vi "LvMPDC_SUB_SendCmdAndRecvReply_2.vi"(6 "timeout_ms":i32=3000, 8 "error in (no error)":errorcluster, 9 "ReadBytes":i32=10240, 10 "Command":string="ping", 11 "Connect ID":refnum<k5>) -> (0 "error out":errorcluster, 2 "Reply":string, 3 "Connect ID out":refnum<k5>)   [LabVIEW 2012]
panel:
  out "Recv String":string
  # "LvMPDC:: Send Command and ReceiveReply"
  # "Replyは、\n末尾の\"OK\\n\"を取り除いた文字列"
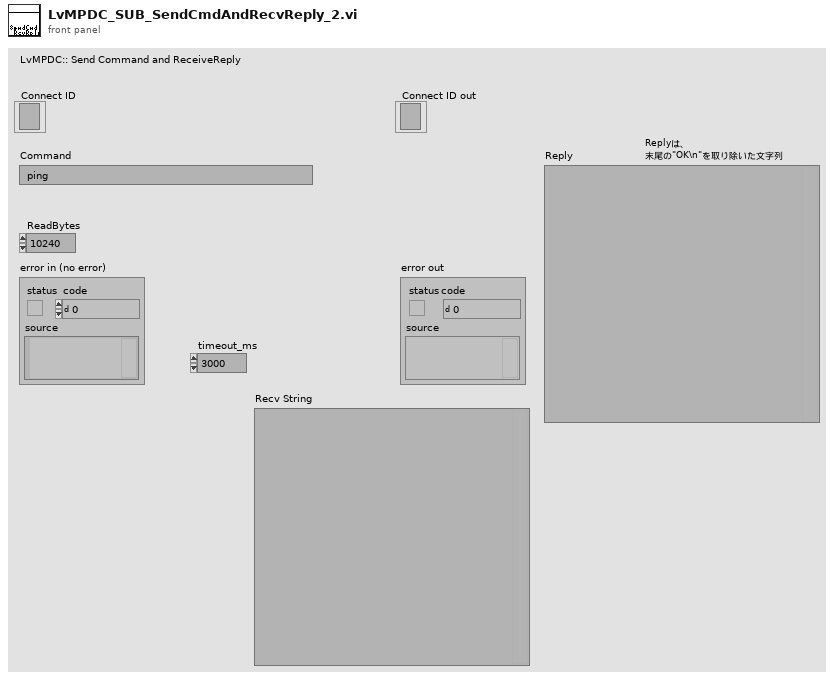
[diagram p1: front panel]
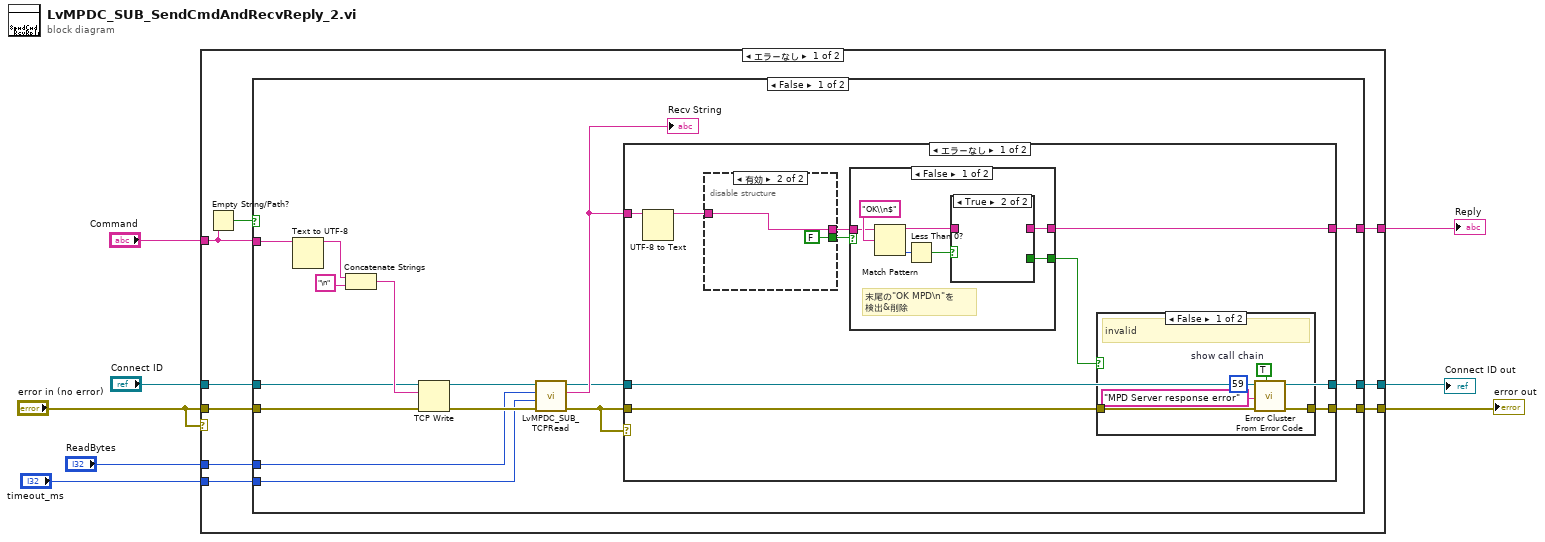
[diagram p0: block diagram]
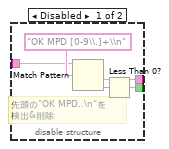
[diagram p2: hidden frame]
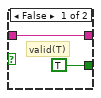
[diagram p4: hidden frame]
diagram:
  n1 = case shown="エラーなし" "error in (no error)" {
    tunnel: "Connect ID" -> [w17 w70]
    tunnel: "error in (no error)" -> [w16 w69]
    tunnel: [w15 w70] -> w7
    tunnel: [w9 w69] -> w6
    tunnel: [w10 _] -> w4
    tunnel: "Command" -> [w14 _]
    tunnel: "timeout_ms" -> [w12 _]
    tunnel: "ReadBytes" -> [w11 _]
    frame No Error {
      n2 = Empty String/Path?(string/path=w14) -> (empty?=w13:bool)
      n3 = case shown="FALSE" w13 {
        tunnel: w17 -> [w29 w68]
        tunnel: w16 -> [w28 w67]
        tunnel: [w19 w68] -> w15
        tunnel: w14 -> [w26 _]
        tunnel: w12 -> [w25 _]
        tunnel: w11 -> [w24 _]
        tunnel: [w22 _] -> w10
        tunnel: [w18 w67] -> w9
        frame False {
          n4 = Text to UTF-8(11:w26) -> (3:w30:string)  [unwired: 1 in, 1 out]
          n5 = Concatenate Strings(w30, "\n" ("データ入力")) -> (w31:string)
          n6 = TCP Write(connection ID=w29, data in=w31, error in (no error)=w28) -> (connection ID out=w33:refnum<k5>, error out=w27:errorcluster)  [unwired: 1 in, 1 out]
          n7 = call "LvMPDC_SUB_TCPRead.vi"("error in (no error)"=w27, "timeout_ms"=w25, "ReadBytes"=w24, "Connect ID"=w33) -> ("error out"=w20:errorcluster, "Recv String"=w23:string, "Connect ID out"=w21:refnum<k5>)  [unwired: 5 in]
          "Recv String" <- w23
          n8 = case shown="エラーなし" w20 {
            tunnel: w23 -> [w34 _]
            tunnel: [w39 _] -> w22
            tunnel: w21 -> [w38 w66]
            tunnel: w20 -> [w36 w65]
            tunnel: [w38 w66] -> w19
            tunnel: [w35 w65] -> w18
            frame No Error {
              n9 = UTF-8 to Text(11:w34) -> (3:w41:string)  [unwired: 1 in, 1 out]
              n10 = disable-structure shown="有効" {
                disable-tunnel: [w46 w49] -> w42
                disable-tunnel: w41 -> [w45 w49]
                disable-tunnel: [w43 FALSE] -> w40
                frame Disabled {
                  # "先頭の\"OK MPD..\\n\"を\n検出&削除"
                  n11 = Match Pattern(string=w45, regular expression="OK MPD [0-9\\.]+\\n" ("正規表現")) -> (after substring=w46:string, offset past match=w44:i32)  [unwired: 1 in, 2 out]
                  n12 = Less Than 0?(x=w44) -> (x < 0?=w43:bool)
                }
                frame Enabled {
                }
              }
              n13 = case shown="FALSE" w40 {
                tunnel: w42 -> [w61 _]
                tunnel: [w57 _] -> w39
                tunnel: [w56 _] -> w37
                frame False {
                  # "末尾の\"OK MPD\\n\"を\n検出&削除"
                  n14 = Match Pattern(string=w61, regular expression="OK\\n$" ("正規表現")) -> (before substring=w58:string, offset past match=w60:i32)  [unwired: 1 in, 2 out]
                  n15 = Less Than 0?(x=w60) -> (x < 0?=w59:bool)
                  n16 = case shown="TRUE" w59 {
                    tunnel: w58 -> [w63 _]
                    tunnel: [w63 _] -> w57
                    tunnel: [TRUE _] -> w56
                    frame False {
                      # "valid(T)"
                    }
                    frame True {
                    }
                  }
                }
                frame True {
                }
              }
              n17 = case shown="FALSE" w37 {
                tunnel: w36 -> [w53 w55]
                tunnel: [w52 w55] -> w35
                frame False {
                  w54 = TRUE  # show call chain
                  # "invalid"
                  n18 = call <vilib>:"Error Cluster From Error Code.vi"("show call chain? (False)"=w54, "error in (no error)"=w53, "error message (\"\")"="MPD Server response error", "error code (0)"=59) -> ("error out"=w52:errorcluster)  [unwired: 5 in]
                }
                frame True {
                  # "valid"
                }
              }
            }
            frame Error {
              # "1文字も受信しなかった場合だけTimeoutエラー"
            }
          }
        }
        frame True {
        }
      }
    }
    frame Error {
    }
  }
  "Connect ID out" <- w7
  "error out" <- w6
  "Reply" <- w4
